vi "Read currentRotatorPositions.vi"(8 "error in (no error)":errorcluster, 11 "PointingPositions in":refnum<class "PointingPositions.lvclass">) -> (0 "error out":errorcluster, 2 "CurrentRotatorPositions.lvclass":refnum<class "CurrentRotatorPositions.lvclass">, 3 "PointingPositions out":refnum<class "PointingPositions.lvclass">)   [LabVIEW 2022 SP3, in "TCSDataDefinitions.lvlib" / "TCSPublicStatus.lvlib" / "PointingPositions.lvlib" / "PointingPositions.lvclass"]
uses:
  PointingPositions.lvclass
  CurrentRotatorPositions/CurrentRotatorPositions.lvclass
  PointingPositions.lvclass/PointingPositions.ctl
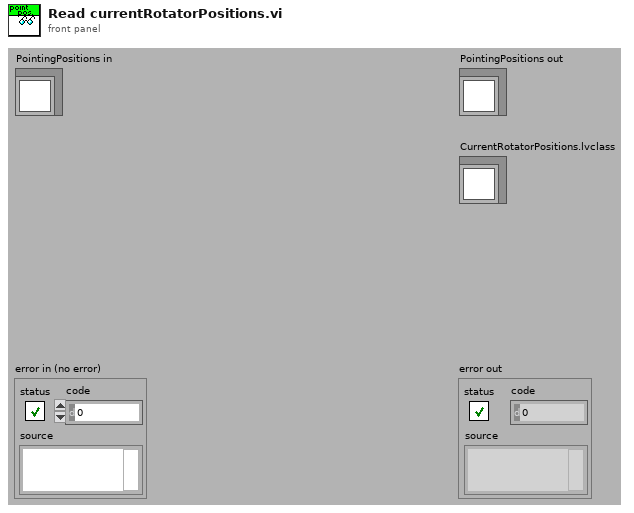
[diagram p1: front panel]
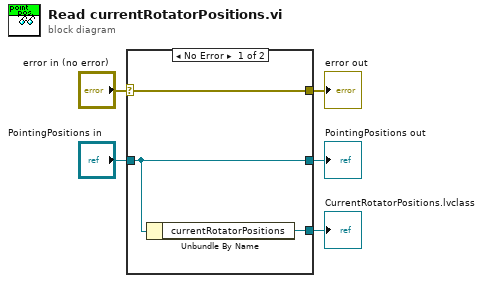
[diagram p0: block diagram]
diagram:
  n1 = case shown="No Error" "error in (no error)" {
    selector: "error in (no error)" -> [w8 w9]
    tunnel: [w8 w9] -> w4
    tunnel: [w7 w10] -> w2
    tunnel: "PointingPositions in" -> [w7 w10]
    tunnel: [w6 _] -> w1
    frame No Error {
      n2 = Unbundle By Name(w7) -> ("currentRotatorPositions"=w6:refnum<class "CurrentRotatorPositions.lvclass">)
    }
    frame Error {
    }
  }
  "error out" <- w4
  "PointingPositions out" <- w2
  "CurrentRotatorPositions.lvclass" <- w1
